vi "Transmitter_Statistics.vi"(6 "Write ?":bool, 8 "error in (no error)":errorcluster, 9 "Frame ID":u32, 10 "Node ID":u32, 11 "Initialize ?":bool) -> (0 "error out":errorcluster, 1 "Start Time (ms)":u32, 2 "Output":T1, 3 "Transmit Packet Data":T1[](array[typedef]))   [LabVIEW 2017]
uses:
  Controls/ADCP_UI/ADCP_UI_Data_Packet_Transmitter_Parameters.ctl
  Controls/ADCP_UI/ADCP_UI_Data_Packet_Receiver_Parameters.ctl
panel:
  out "Execution time (ms)":u32
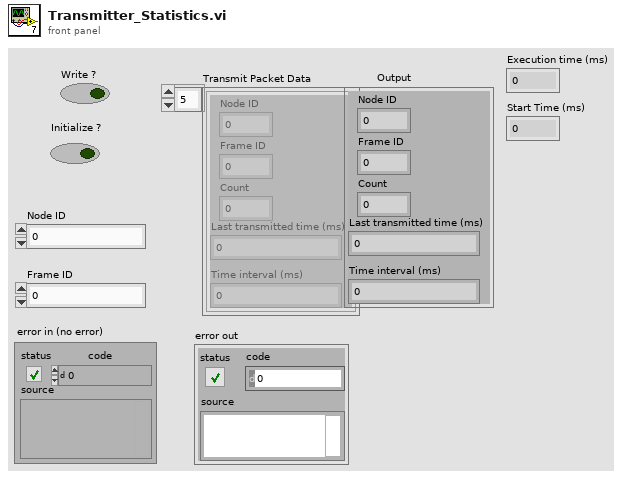
[diagram p1: front panel]
types:
  T1 = typedef "ADCP_UI_Data_Packet_Transmitter_Parameters.ctl" = cluster{"Node ID":u32, "Frame ID":u32, "Count":u32, "Last transmitted time (ms)":u32, "Time interval (ms)":u32}
  T2 = typedef "ADCP_UI_Data_Packet_Receiver_Parameters.ctl" = cluster{"Node ID":u32, "Frame ID":u32, "Count":u32, "Last received time (ms)":u32, "Time interval (ms)":u32}
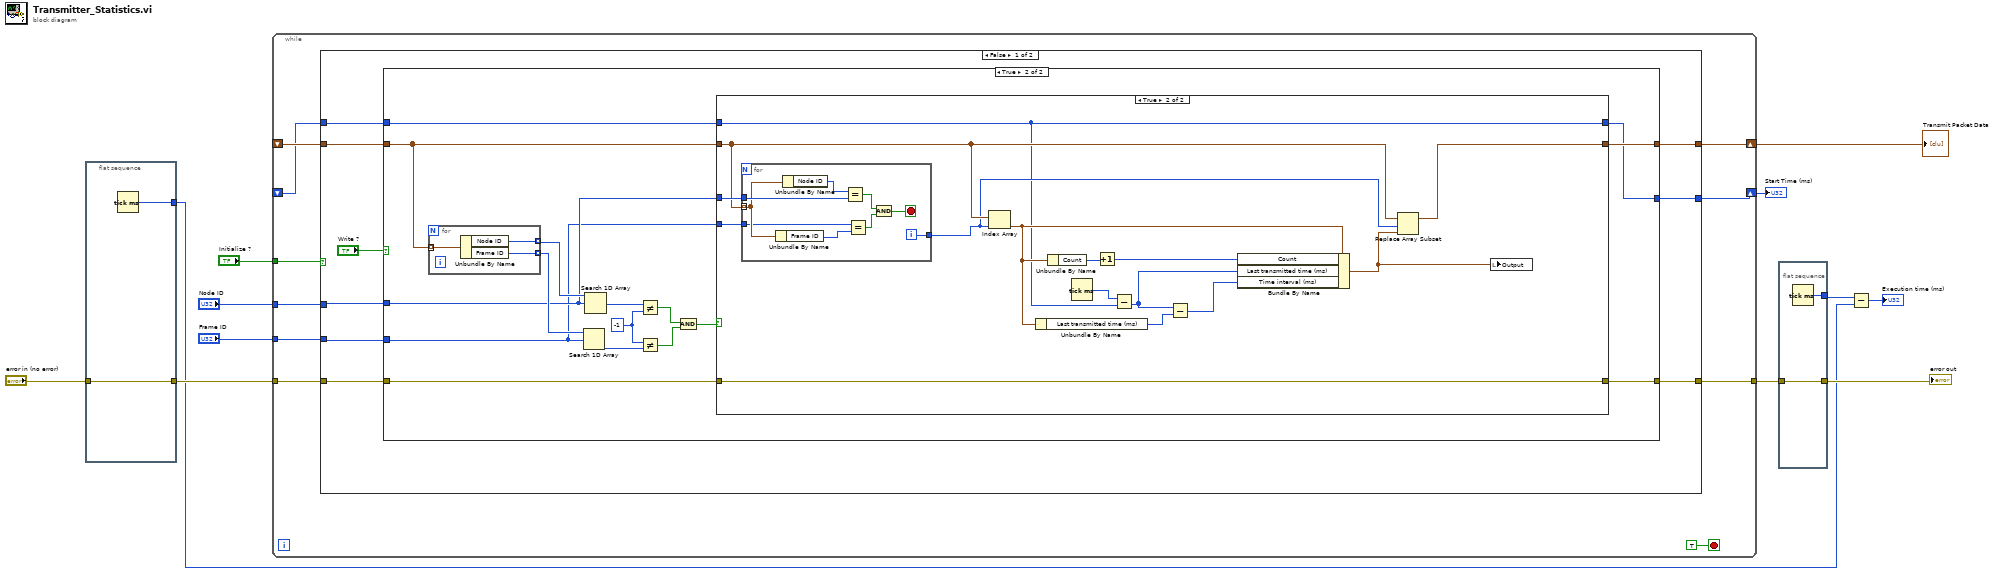
[diagram p0: block diagram]
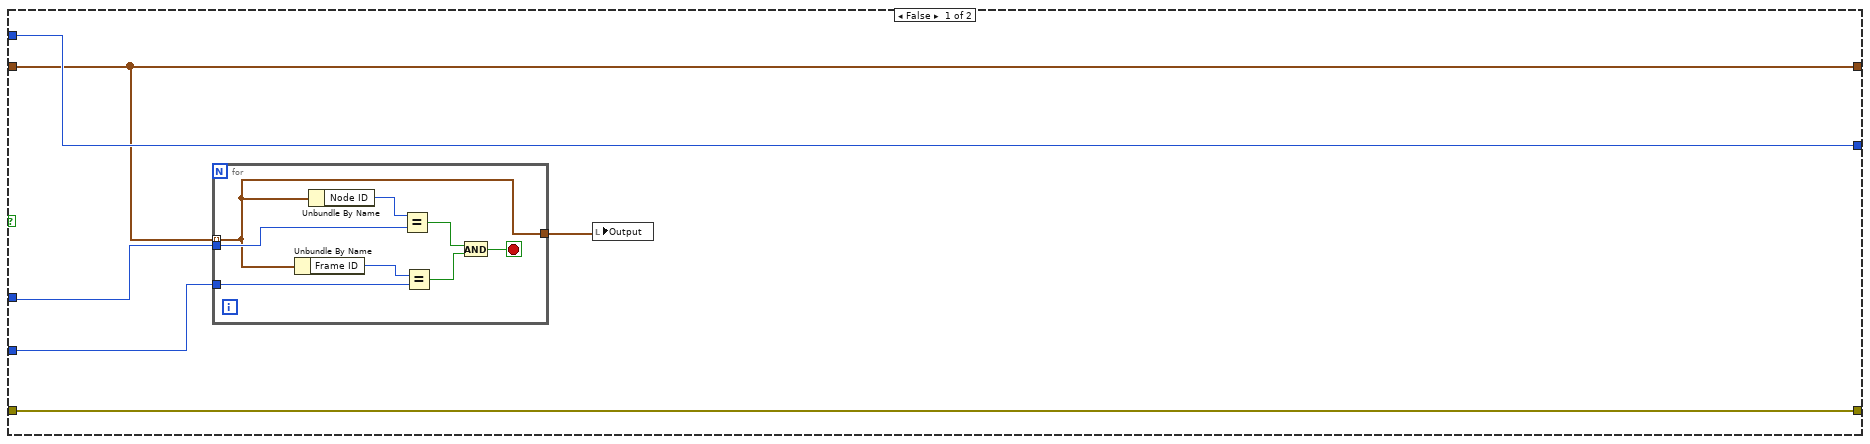
[diagram p2: hidden frame]
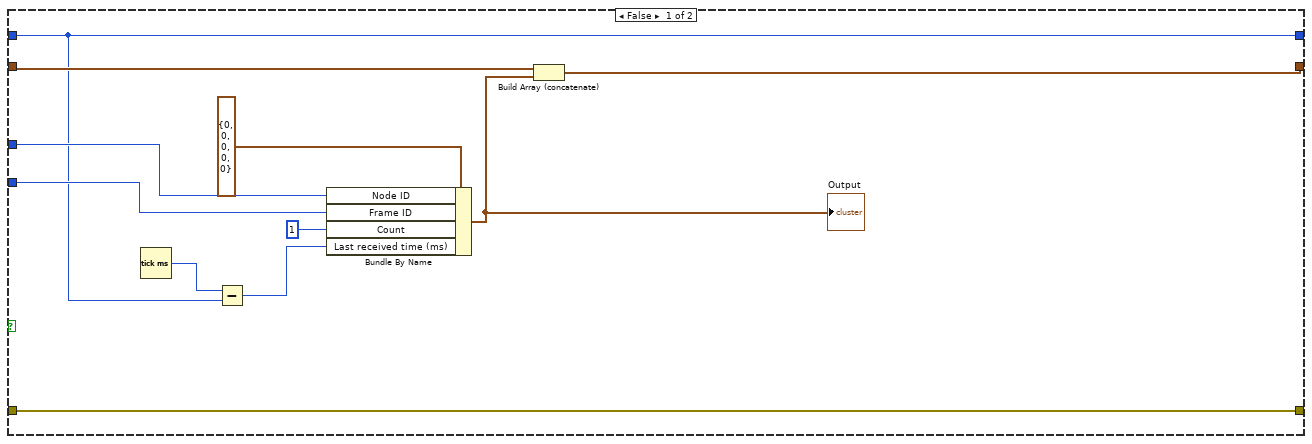
[diagram p3: hidden frame]
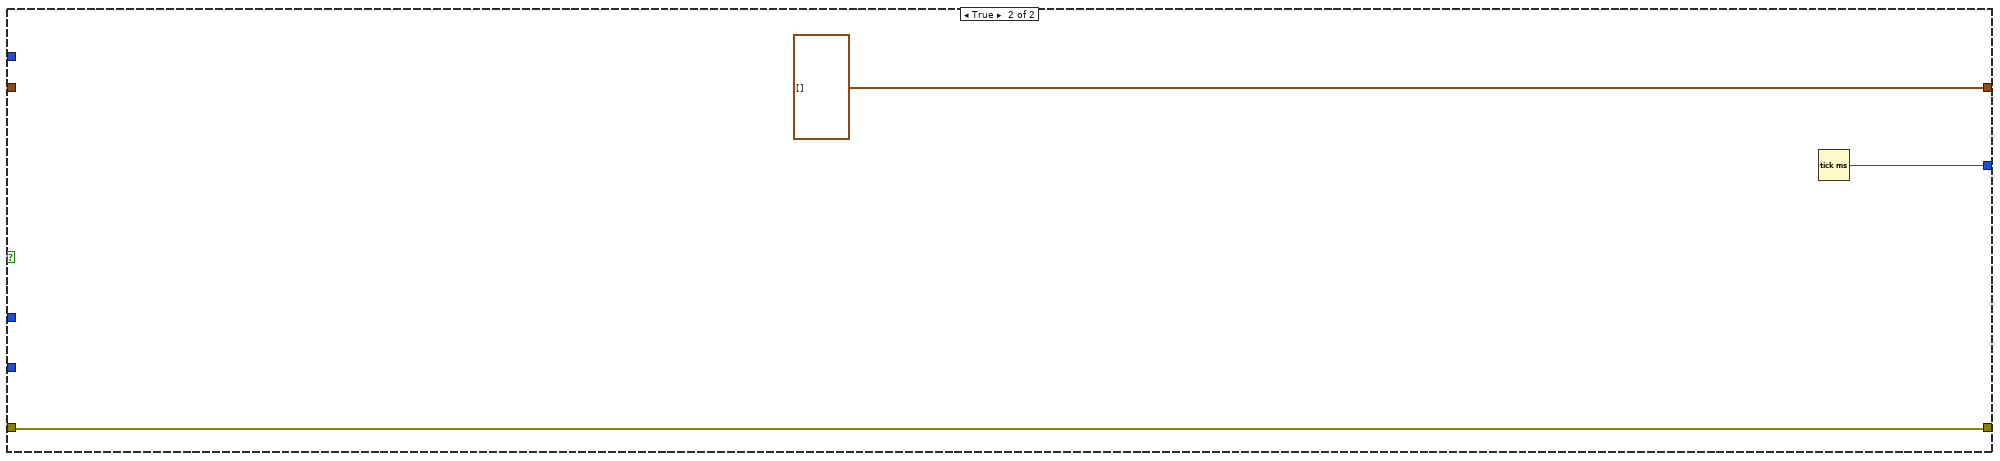
[diagram p4: hidden frame]
diagram:
  n1 = flat-sequence {
    tunnel: "error in (no error)" -> [w14]
    tunnel: [w14] -> w7
    tunnel: [w13] -> w3
    frame #0 {
      n2 = Tick Count (ms)() -> (millisecond timer value=w13:u32)
    }
  }
  n3 = while {
    tunnel: w7 -> [w23]
    tunnel: "Initialize ?" -> [w22]
    tunnel: "Node ID" -> [w21]
    tunnel: "Frame ID" -> [w20]
    shift-right: [w19] -> w9
    shift-left: _ -> [w18]
    tunnel: [w17] -> w6
    shift-right: [w16] -> w1
    shift-left: _ -> [w15]
    stop <- TRUE stop-if-true
    n4 = case shown="False" w22 {
      tunnel: w23 -> [w29 w103]
      tunnel: w21 -> [w32 _]
      tunnel: w20 -> [w31 _]
      tunnel: [w30 T1[] []] -> w19
      tunnel: w18 -> [w33 _]
      tunnel: [w28 w103] -> w17
      tunnel: [w26 w102] -> w16
      tunnel: w15 -> [w27 _]
      frame False {
        n5 = case shown="True" "Write ?" {
          tunnel: w33 -> [w37 w55]
          tunnel: w32 -> [w36 w54]
          tunnel: w31 -> [w35 w53]
          tunnel: [w37 w52] -> w30
          tunnel: w29 -> [w39 w51]
          tunnel: [w39 w50] -> w28
          tunnel: w27 -> [w38 w49]
          tunnel: [w38 w48] -> w26
          frame False {
            n6 = for {
              tunnel: w37 -> [w41] mode=indexing
              tunnel: w36 -> [w46]
              tunnel: w35 -> [w44]
              tunnel: [w41] -> w34
              stop <- w40 stop-if-true
              n7 = Unbundle By Name(w41) -> ("Frame ID"=w45:u32)
              n8 = Unbundle By Name(w41) -> ("Node ID"=w47:u32)
              n9 = Equal?(x=w47, y=w46) -> (x = y?=w43:bool)
              n10 = Equal?(x=w45, y=w44) -> (x = y?=w42:bool)
              n11 = And(x=w43, y=w42) -> (x .and. y?=w40:bool)
            }
            n12 = local write "Output"(w34) -> ()
          }
          frame True {
            w59 = -1 ("y")
            n13 = for {
              tunnel: w55 -> [w101] mode=indexing
              tunnel: [w100] -> w63 mode=indexing
              tunnel: [w99] -> w62 mode=indexing
              n14 = Unbundle By Name(w101) -> ("Node ID"=w100:u32, "Frame ID"=w99:u32)
            }
            n15 = Search 1D Array(1D array=w62, element=w53) -> (index of element=w60:i32)  [unwired: 1 in]
            n16 = Search 1D Array(1D array=w63, element=w54) -> (index of element=w61:i32)  [unwired: 1 in]
            n17 = Not Equal?(x=w59, y=w60) -> (x != y?=w57:bool)
            n18 = Not Equal?(x=w61, y=w59) -> (x != y?=w58:bool)
            n19 = And(x=w58, y=w57) -> (x .and. y?=w56:bool)
            n20 = case shown="True" w56 {
              tunnel: w55 -> [w71 w85]
              tunnel: w54 -> [w74 w89]
              tunnel: w53 -> [w73 w88]
              tunnel: [w70 w83] -> w52
              tunnel: w51 -> [w69 w82]
              tunnel: [w69 w82] -> w50
              tunnel: w49 -> [w64 w76]
              tunnel: [w64 w76] -> w48
              frame False {
                n21 = Tick Count (ms)() -> (millisecond timer value=w66:u32)
                n22 = Subtract(x=w66, y=w64) -> (x-y=w65:u32)
                n23 = Bundle By Name(cluster=T2 {"Node ID"=0, "Frame ID"=0, "Count"=0, "Last received time (ms)"=0, "Time interval (ms)"=0} ("Cluster"), "Node ID"=w74, "Frame ID"=w73, "Count"=u32 1, "Last received time (ms)"=w65) -> (w67:T2)
                "Output" <- w67
                n24 = Build Array (concatenate)(w71, w67) -> (w70:T2[])
              }
              frame True {
                n25 = for {
                  tunnel: w85 -> [w96] mode=indexing
                  tunnel: w89 -> [w97]
                  tunnel: w88 -> [w94]
                  tunnel: [w90] -> w84
                  i -> [w90]
                  stop <- w91 stop-if-true
                  n26 = Unbundle By Name(w96) -> ("Frame ID"=w95:u32)
                  n27 = Unbundle By Name(w96) -> ("Node ID"=w98:u32)
                  n28 = Equal?(x=w98, y=w97) -> (x = y?=w92:bool)
                  n29 = Equal?(x=w94, y=w95) -> (x = y?=w93:bool)
                  n30 = And(x=w92, y=w93) -> (x .and. y?=w91:bool)
                }
                n31 = Index Array(array=w85, index=w84) -> (element=w80:T1)
                n32 = Unbundle By Name(w80) -> ("Last transmitted time (ms)"=w79:u32)
                n33 = Unbundle By Name(w80) -> ("Count"=w87:u32)
                n34 = Tick Count (ms)() -> (millisecond timer value=w77:u32)
                n35 = Increment(x=w87) -> (x+1=w86:u32)
                n36 = Subtract(x=w77, y=w76) -> (x-y=w75:u32)
                n37 = Subtract(x=w75, y=w79) -> (x-y=w78:u32)
                n38 = Bundle By Name(cluster=w80, "Count"=w86, "Last transmitted time (ms)"=w75, "Time interval (ms)"=w78) -> (w81:T1)
                n39 = Replace Array Subset(array=w85, new element=w81, index=w84) -> (w83:T1[])
                n40 = local write "Output"(w81) -> ()
              }
            }
          }
        }
      }
      frame True {
        n41 = Tick Count (ms)() -> (millisecond timer value=w102:u32)
      }
    }
  }
  "Transmit Packet Data" <- w9
  "Start Time (ms)" <- w1
  n42 = flat-sequence {
    tunnel: w6 -> [w106]
    tunnel: [w106] -> w5
    tunnel: [w105] -> w4
    frame #0 {
      n43 = Tick Count (ms)() -> (millisecond timer value=w105:u32)
    }
  }
  n44 = Subtract(x=w4, y=w3) -> (x-y=→"Execution time (ms)":u32)
  "error out" <- w5
